vi "Begin.vi"(8 "error in":errorcluster) -> (0 "error out":errorcluster)   [LabVIEW 2018]
doc: "Called before other user functions, this VI is expected to open initial I/O refnums, load in file data, and do all program initialization. Notice that the <B>error out</B> terminal is simply used for data flow. Wiring it to other structures or subVIs ensures that this VI runs first."
uses:
  <vilib>/Rock Robotics/WPI/ThirdParty/Phoenix-LabVIEW/Motor Controller/Controls/CTRE_Phoenix_MotorControl_EnhancedMotorControllerConfigurables.ctl
  <vilib>/Rock Robotics/WPI/ThirdParty/Phoenix-LabVIEW/Motor Controller/Controls/CTRE_Phoenix_MotorControl_BaseConfigurables.ctl
  <vilib>/Rock Robotics/WPI/ThirdParty/Phoenix-LabVIEW/Motor Controller/Controls/CTRE_Phoenix_MotorControl_VelocityMeasurementPeriod.ctl
  <vilib>/Rock Robotics/WPI/ThirdParty/Phoenix-LabVIEW/Motor Controller/Controls/CTRE_Phoenix_MotorControl_SlotStructure.ctl
  <vilib>/Rock Robotics/WPI/ThirdParty/Phoenix-LabVIEW/Motor Controller/Controls/CTRE_Phoenix_MotorControl_FilterStruct.ctl
  <vilib>/Rock Robotics/WPI/ThirdParty/Phoenix-LabVIEW/Motor Controller/Controls/CTRE_Phoenix_MotorControl_RemoteSourceType.ctl
  <vilib>/Rock Robotics/WPI/ThirdParty/Phoenix-LabVIEW/Controls/CTRE_Phoenix_CustomParamConfiguration.ctl
  <vilib>/Rock Robotics/WPI/ThirdParty/Phoenix-LabVIEW/Motor Controller/Controls/CTRE_Phoenix_MotorControl_FeedbackDevice.ctl
  <vilib>/Rock Robotics/WPI/ThirdParty/Phoenix-LabVIEW/Motor Controller/Controls/CTRE_Phoenix_MotorControl_SensorTermFeedbackDevice_Enhanced.ctl
  <vilib>/Rock Robotics/WPI/ThirdParty/Phoenix-LabVIEW/Motor Controller/Controls/CTRE_Phoenix_MotorControl_LimitSwitchNormal.ctl
  <vilib>/Rock Robotics/WPI/ThirdParty/Phoenix-LabVIEW/Motor Controller/Controls/CTRE_Phoenix_MotorControl_LimitSwitchSource_Local.ctl
  <vilib>/Rock Robotics/WPI/ThirdParty/Phoenix-LabVIEW/Motor Controller/Controls/CTRE_Phoenix_MotorControl_MotorControllerConfigurables.ctl
  <vilib>/Rock Robotics/WPI/ThirdParty/Phoenix-LabVIEW/Motor Controller/Controls/CTRE_Phoenix_MotorControl_RemoteFeedbackDevice.ctl
  <vilib>/Rock Robotics/WPI/ThirdParty/Phoenix-LabVIEW/Motor Controller/Controls/CTRE_Phoenix_MotorControl_SensorTermFeedbackDevice.ctl
  <vilib>/Rock Robotics/WPI/ThirdParty/Phoenix-LabVIEW/Motor Controller/Controls/CTRE_Phoenix_MotorControl_LimitSwitchSource.ctl
  <vilib>/Rock Robotics/WPI/DriverStation/WPI_DriverStationRobotMode2.ctl
  <vilib>/Rock Robotics/WPI/Joystick/WPI_JoystickDeviceEnum.ctl
  <vilib>/Rock Robotics/WPI/Solenoid/WPI_SolenoidChannel.ctl
  <vilib>/Rock Robotics/SystemInterfaces/AI/FPGA_AIChannel.ctl
  <vilib>/Rock Robotics/WPI/ThirdParty/Phoenix-LabVIEW/Motor Controller/Controls/CTRE_Phoenix_MotorControl_NeutralMode.ctl
  <vilib>/Rock Robotics/WPI/SafetyOutput/WPI_SafetyOutputConfigMenu.ctl
  <vilib>/Rock Robotics/WPI/Accelerometer/WPI_AccelerometerRange.ctl
  <vilib>/Rock Robotics/WPI/ThirdParty/REV Robotics/SPARK MAX/Typedef/Spark MAX Idle Mode.ctl
  <vilib>/Rock Robotics/SystemInterfaces/DIO/FPGA_DIOPWMChannel.ctl
  Robot Global Data.vi
  RefNums_DriverStation.vi
  <vilib>/Rock Robotics/Network Tables/NT Write String Array.vi
  <vilib>/Rock Robotics/WPI/Solenoid/WPI_SolenoidOpenDouble.vi
  RefNums_Actuators.vi
  <vilib>/Rock Robotics/WPI/Utilities/WPI_GetSetVariantRefNum.vi
  RefNums_Sensors.vi
  <vilib>/Rock Robotics/WPI/Accelerometer/InternalAccelerometer/WPI_AccelerometerInternalOpen.vi
  <vilib>/Rock Robotics/WPI/Solenoid/WPI_SolenoidOpenSingle.vi
  <vilib>/Rock Robotics/WPI/RobotDrive/WPI_RobotDriveOpen4MotorWithExistingMotors.vi
panel:
  in  "Victor Enhanced Control":T1={"Base Configurables"={"openLoopRamp"=0.0, "closedLoopRamp"=0.0, "peakOutputForward"=1.0, "peakOutputReverse"=-1.0, "nominalOutputForward"=0.0, "nominalOutputReverse"=0.0, "neutralDeadband"=0.04, "voltageCompSaturation"=0.0, "voltageMeasurementFilter"=32, "velocityMeasurementPeriod"=100, "velocityMeasurementWindow"=64, "forwardSoftLimitThreshold"=0, "reverseSoftLimitThreshold"=0, "forwardSoftLimitEnable"=FALSE, "reverseSoftLimitEnable"=FALSE, "slot0"={"P"=0.0, "I"=0.0, "D"=0.0, "F"=0.0, "integralZone"=0.0, "allowableClosedLoopError"=0, "maxIntegralAccumulator"=0.0, "closedLoopPeakOutput"=1.0, "closedLoopPeriod"=1}, "slot1"={"P"=0.0, "I"=0.0, "D"=0.0, "F"=0.0, "integralZone"=0.0, "allowableClosedLoopError"=0, "maxIntegralAccumulator"=0.0, "closedLoopPeakOutput"=1.0, "closedLoopPeriod"=1}, "slot2"={"P"=0.0, "I"=0.0, "D"=0.0, "F"=0.0, "integralZone"=0.0, "allowableClosedLoopError"=0, "maxIntegralAccumulator"=0.0, "closedLoopPeakOutput"=1.0, "closedLoopPeriod"=1}, "slot3"={"P"=0.0, "I"=0.0, "D"=0.0, "F"=0.0, "integralZone"=0.0, "allowableClosedLoopError"=0, "maxIntegralAccumulator"=0.0, "closedLoopPeakOutput"=1.0, "closedLoopPeriod"=1}, "auxPIDPolarity"=FALSE, "remoteFilter0"={"remoteSensorDeviceID"=0, "remoteSensorSource"=enum."Off"}, "remoteFilter1"={"remoteSensorDeviceID"=0, "remoteSensorSource"=enum."Off"}, "motionCruiseVelocity"=0, "motionAcceleration"=0, "motionProfileTrajectoryPeriod"=0, "feedbackNotContinuous"=FALSE, "remoteSensorClosedLoopDisableNeutralOnLOS"=FALSE, "clearPositionOnLimitF"=FALSE, "clearPositionOnLimitR"=FALSE, "clearPositionOnQuadIdx"=FALSE, "limitSwitchDisableNeutralOnLOS"=FALSE, "softLimitDisableNeutralOnLOS"=FALSE, "pulseWidthPeriod_EdgesPerRot"=1, "pulseWidthPeriod_FilterWindowSz"=1, "customParam"={"customParam0"=0, "customParam1"=0}, "trajectoryInterpolationEnable"=TRUE}, "primaryPID"={"selectedFeedbackCoefficient"=1.0, "selectedFeedbackSensor"=11}, "auxiliaryPID"={"selectedFeedbackCoefficient"=1.0, "selectedFeedbackSensor"=11}, "sum 0 term"=11, "sum 1 term"=11, "diff 0 term "=11, "diff 1 term"=11, "forwardLimitSwitchDeviceID"=0, "reverseLimitSwitchDeviceID"=0, "forwardLimitSwitchNormal"=enum."Normally Open", "reverseLimitSwitchNormal"=enum."Normally Open", "forwardLimitSwitchSource"=3, "reverseLimitSwitchSource"=3} {"diff 1 term" items=["Remote Source 0"=11, "Remote Source 1"=12, "Software Emulated"=15]; "diff 0 term" items=["Remote Source 0"=11, "Remote Source 1"=12, "Software Emulated"=15]; "sum 1 term" items=["Remote Source 0"=11, "Remote Source 1"=12, "Software Emulated"=15]; "sum 0 term" items=["Remote Source 0"=11, "Remote Source 1"=12, "Software Emulated"=15]; "reverseLimitSwitchSource" items=["Remote Talon SRX"=1, "Remote CANifier"=2, "Deactivated"=3]; "forwardLimitSwitchSource" items=["Remote Talon SRX"=1, "Remote CANifier"=2, "Deactivated"=3]; "auxiliaryPID"."selectedFeedbackSensor" items=["Sensor Sum (S0 + S1)"=9, "Sensor Difference (D0 - D1)"=10, "Remote Source 0"=11, "Remote Source 1"=12, "Software Emulated"=15]; "primaryPID"."selectedFeedbackSensor" items=["Sensor Sum (S0 + S1)"=9, "Sensor Difference (D0 - D1)"=10, "Remote Source 0"=11, "Remote Source 1"=12, "Software Emulated"=15]; "Base Configurables"."velocityMeasurementPeriod" items=["Period_1ms"=1, "Period_2ms"=2, "Period_5ms"=5, "Period_10ms"=10, "Period_20ms"=20, "Period_25ms"=25, "Period_50ms"=50, "Period_100ms"=100]}
  in  "Talon Enhanced Config":T12={"Base Configurables"={"openLoopRamp"=0.0, "closedLoopRamp"=0.0, "peakOutputForward"=1.0, "peakOutputReverse"=-1.0, "nominalOutputForward"=0.0, "nominalOutputReverse"=0.0, "neutralDeadband"=0.04, "voltageCompSaturation"=0.0, "voltageMeasurementFilter"=32, "velocityMeasurementPeriod"=100, "velocityMeasurementWindow"=64, "forwardSoftLimitThreshold"=0, "reverseSoftLimitThreshold"=0, "forwardSoftLimitEnable"=FALSE, "reverseSoftLimitEnable"=FALSE, "slot0"={"P"=0.0, "I"=0.0, "D"=0.0, "F"=0.0, "integralZone"=0.0, "allowableClosedLoopError"=0, "maxIntegralAccumulator"=0.0, "closedLoopPeakOutput"=1.0, "closedLoopPeriod"=1}, "slot1"={"P"=0.0, "I"=0.0, "D"=0.0, "F"=0.0, "integralZone"=0.0, "allowableClosedLoopError"=0, "maxIntegralAccumulator"=0.0, "closedLoopPeakOutput"=1.0, "closedLoopPeriod"=1}, "slot2"={"P"=0.0, "I"=0.0, "D"=0.0, "F"=0.0, "integralZone"=0.0, "allowableClosedLoopError"=0, "maxIntegralAccumulator"=0.0, "closedLoopPeakOutput"=1.0, "closedLoopPeriod"=1}, "slot3"={"P"=0.0, "I"=0.0, "D"=0.0, "F"=0.0, "integralZone"=0.0, "allowableClosedLoopError"=0, "maxIntegralAccumulator"=0.0, "closedLoopPeakOutput"=1.0, "closedLoopPeriod"=1}, "auxPIDPolarity"=FALSE, "remoteFilter0"={"remoteSensorDeviceID"=0, "remoteSensorSource"=enum."Off"}, "remoteFilter1"={"remoteSensorDeviceID"=0, "remoteSensorSource"=enum."Off"}, "motionCruiseVelocity"=0, "motionAcceleration"=0, "motionProfileTrajectoryPeriod"=0, "feedbackNotContinuous"=FALSE, "remoteSensorClosedLoopDisableNeutralOnLOS"=FALSE, "clearPositionOnLimitF"=FALSE, "clearPositionOnLimitR"=FALSE, "clearPositionOnQuadIdx"=FALSE, "limitSwitchDisableNeutralOnLOS"=FALSE, "softLimitDisableNeutralOnLOS"=FALSE, "pulseWidthPeriod_EdgesPerRot"=1, "pulseWidthPeriod_FilterWindowSz"=1, "customParam"={"customParam0"=0, "customParam1"=0}, "trajectoryInterpolationEnable"=TRUE}, "primaryPID"={"selectedFeedbackCoefficient"=1.0, "selectedFeedbackSensor"=0}, "auxiliaryPID"={"selectedFeedbackCoefficient"=1.0, "selectedFeedbackSensor"=0}, "sum0Term"=0, "sum1Term"=0, "diff0Term"=0, "diff1Term"=0, "forwardLimitSwitchNormal"=enum."Normally Open", "reverseLimitSwitchNormal"=enum."Normally Open", "forwardLimitSwitchDeviceID"=0, "reverseLimitSwitchDeviceID"=0, "forwardLimitSwitchSource"=enum."Feedback Connector", "reverseLimitSwitchSource"=enum."Feedback Connector", "peakCurrentLimit"=1, "peakCurrentDuration"=1, "continuousCurrentLimit"=1} {"diff1Term" items=["QuadEncoder"=0, "Analog"=2, "Tachometer"=4, "Pulse Width Encoded Position"=8, "Remote Source 0"=11, "Remote Source 1"=12, "Software Emulated"=15]; "diff0Term" items=["QuadEncoder"=0, "Analog"=2, "Tachometer"=4, "Pulse Width Encoded Position"=8, "Remote Source 0"=11, "Remote Source 1"=12, "Software Emulated"=15]; "sum1Term" items=["QuadEncoder"=0, "Analog"=2, "Tachometer"=4, "Pulse Width Encoded Position"=8, "Remote Source 0"=11, "Remote Source 1"=12, "Software Emulated"=15]; "sum0Term" items=["QuadEncoder"=0, "Analog"=2, "Tachometer"=4, "Pulse Width Encoded Position"=8, "Remote Source 0"=11, "Remote Source 1"=12, "Software Emulated"=15]; "auxiliaryPID"."selectedFeedbackSensor" items=["QuadEncoder"=0, "Analog"=2, "Tachometer"=4, "Pulse Width Encoded Position"=8, "Sensor Sum (S0 + S1)"=9, "Sensor Difference (D0 - D1)"=10, "Remote Source 0"=11, "Remote Source 1"=12, "Software Emulated"=15]; "primaryPID"."selectedFeedbackSensor" items=["QuadEncoder"=0, "Analog"=2, "Tachometer"=4, "Pulse Width Encoded Position"=8, "Sensor Sum (S0 + S1)"=9, "Sensor Difference (D0 - D1)"=10, "Remote Source 0"=11, "Remote Source 1"=12, "Software Emulated"=15]; "Base Configurables"."velocityMeasurementPeriod" items=["Period_1ms"=1, "Period_2ms"=2, "Period_5ms"=5, "Period_10ms"=10, "Period_20ms"=20, "Period_25ms"=25, "Period_50ms"=50, "Period_100ms"=100]}
  # "Sum and Diff terms are ways to select more than one sensor as a feedback device. \n Sum 0 is the first feedback device to be used for the Sum term, \n Sum 1 is the feedback device to be added to Sum 0 for the Sum term\n Diff 0 and Diff 1 work in a similar manner"
  # "These are only applicable\nif using a remote limit switch.\n\nLocal limit switches/no limit\nswitches do not use this"
  # "False: Primary Output = PID[0] + PID[1]  ---  Auxiliary Output = PID[0] - PID[1]\nTrue:  Primary Output = PID[0] - PID[1] --- Auxiliary Output = PID[0] + PID[1]"
  # "Enable the motion profile executor to perform linear interpolation between profile points.  Defaults to True."
  # "Sum and Diff terms are ways to select more than one sensor as a feedback device. \n Sum 0 is the first feedback device to be used for the Sum term.\n Sum 1 is the feedback device to be added to Sum 0 for the Sum term.\n Diff 0 and Diff 1 work in a similar manner."
  # "These are only applicable\nif using a remote limit switch.\n\nLocal limit switches/no limit\nswitches do not use this."
  # "Current is below Continuous threshold AND\n\n(Requested output is weaker** than applied motor\noutput OR is in the opposite direction).\n/\nMotor output is set to requested output."
  # "Current is above Peak* Threshold for Peak Duration.\n/\nReduce motor output (towards neutral)."
  # "Current is below Continuous threshold.\n/\nRamp motor output towards requested output."
  # "Current is above Continuous threshold.\n/\nReduce motor output (towards neutral)."
  # "Current Limiting is NOT enabled\nby default.\nCall this VI to enable."
  # "*If the configured Peak Threshold is less than the Continuous Threshold, the applied Peak Threshold is set equal to the Configured Continuous Threshold in firmware.\n** Both requested output and applied motor output are in the same direction, and requested output is closer to neutral."
  # "False: Primary Output = PID[0] + PID[1]  ---  Auxiliary Output = PID[0] - PID[1]\nTrue:  Primary Output = PID[0] - PID[1] --- Auxiliary Output = PID[0] + PID[1]"
  # "Enable the motion profile executor to perform linear interpolation between profile points.  Defaults to True."
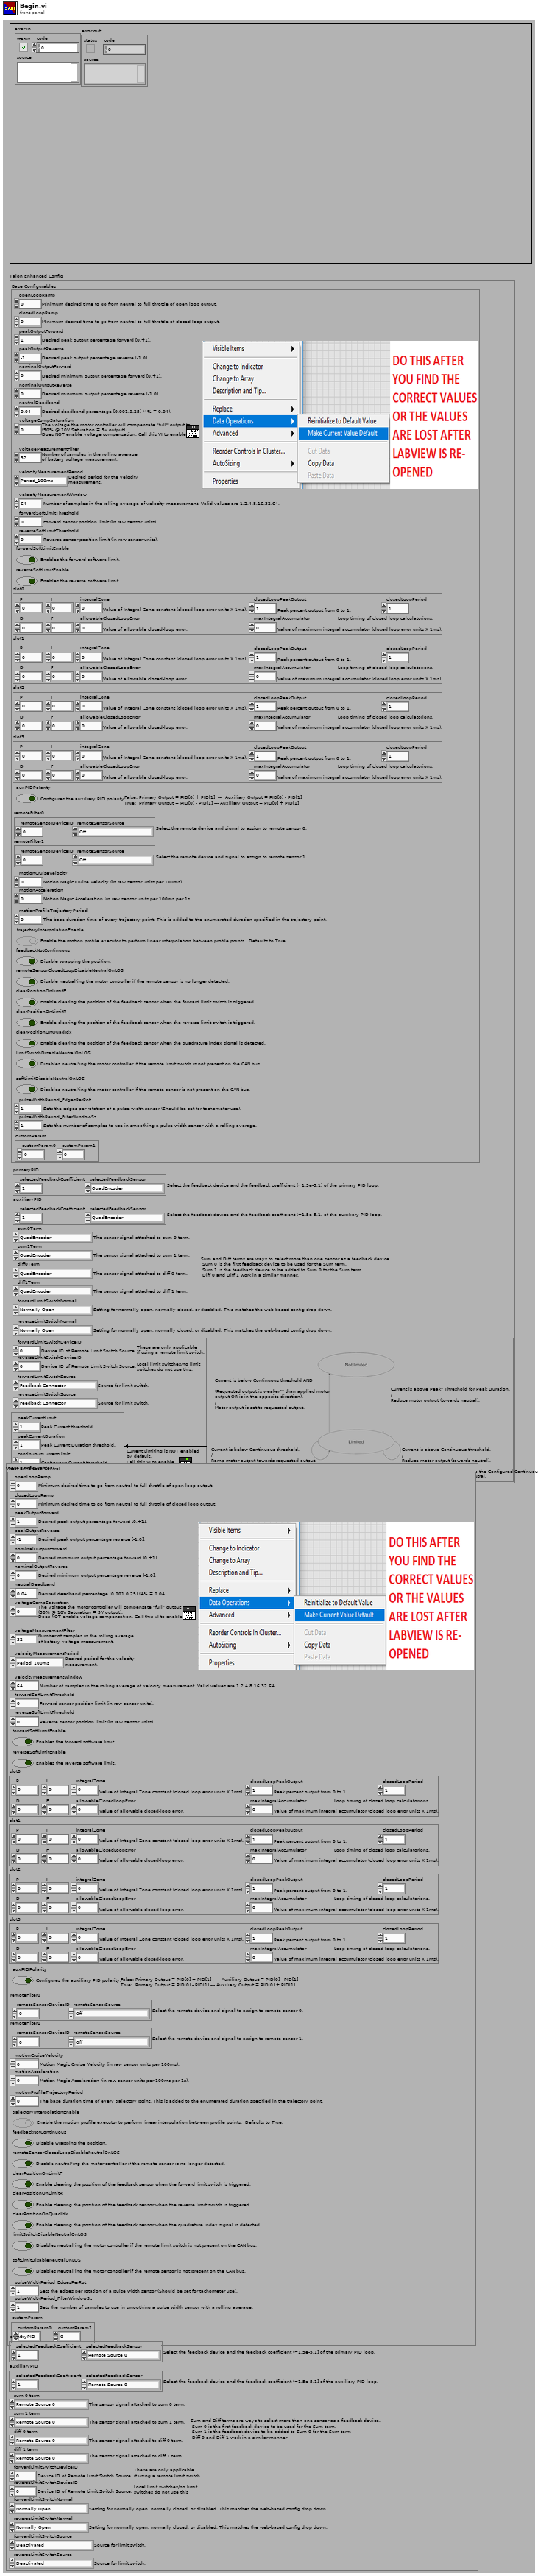
[diagram p1: front panel]
types:
  T1 = typedef "CTRE_Phoenix_MotorControl_MotorControllerConfigurables.ctl" = cluster{"Base Configurables":T2, "primaryPID":cluster{"selectedFeedbackCoefficient":dbl, "selectedFeedbackSensor":T8}, "auxiliaryPID":cluster{"selectedFeedbackCoefficient":dbl, "selectedFeedbackSensor":T8}, "sum 0 term":T9, "sum 1 term":T9, "diff 0 term ":T9, "diff 1 term":T9, "forwardLimitSwitchDeviceID":i32, "reverseLimitSwitchDeviceID":i32, "forwardLimitSwitchNormal":T10, "reverseLimitSwitchNormal":T10, "forwardLimitSwitchSource":T11, "reverseLimitSwitchSource":T11}
  T2 = typedef "CTRE_Phoenix_MotorControl_BaseConfigurables.ctl" = cluster{"openLoopRamp":dbl, "closedLoopRamp":dbl, "peakOutputForward":dbl, "peakOutputReverse":dbl, "nominalOutputForward":dbl, "nominalOutputReverse":dbl, "neutralDeadband":dbl, "voltageCompSaturation":dbl, "voltageMeasurementFilter":i32, "velocityMeasurementPeriod":T3, "velocityMeasurementWindow":i32, "forwardSoftLimitThreshold":i32, "reverseSoftLimitThreshold":i32, "forwardSoftLimitEnable":bool, "reverseSoftLimitEnable":bool, "slot0":T4, "slot1":T4, "slot2":T4, "slot3":T4, "auxPIDPolarity":bool, "remoteFilter0":T5, "remoteFilter1":T5, "motionCruiseVelocity":i32, "motionAcceleration":i32, "motionProfileTrajectoryPeriod":i32, "feedbackNotContinuous":bool, "remoteSensorClosedLoopDisableNeutralOnLOS":bool, "clearPositionOnLimitF":bool, "clearPositionOnLimitR":bool, "clearPositionOnQuadIdx":bool, "limitSwitchDisableNeutralOnLOS":bool, "softLimitDisableNeutralOnLOS":bool, "pulseWidthPeriod_EdgesPerRot":i32, "pulseWidthPeriod_FilterWindowSz":i32, "customParam":T7, "trajectoryInterpolationEnable":bool}
  T3 = typedef "CTRE_Phoenix_MotorControl_VelocityMeasurementPeriod.ctl" = u16
  T4 = typedef "CTRE_Phoenix_MotorControl_SlotStructure.ctl" = cluster{"P":dbl, "I":dbl, "D":dbl, "F":dbl, "integralZone":dbl, "allowableClosedLoopError":i32, "maxIntegralAccumulator":dbl, "closedLoopPeakOutput":dbl, "closedLoopPeriod":i32}
  T5 = typedef "CTRE_Phoenix_MotorControl_FilterStruct.ctl" = cluster{"remoteSensorDeviceID":u8, "remoteSensorSource":T6}
  T6 = typedef "CTRE_Phoenix_MotorControl_RemoteSourceType.ctl" = enum16{"Off", "Talon SRX Selected Sensor", "Pigeon IMU Yaw", "Pigeon IMU Pitch", "Pigeon IMU Roll", "CANifier Quadrature", "CANifier PWM Input 0", "CANifier PWM Input 1", "CANifier PWM Input 2", "CANifier PWM Input 3", "Gadgeteer Pigeon Yaw", "Gadgeteer Pigeon Pitch", "Gadgeteer Pigeon Roll"}
  T7 = typedef "CTRE_Phoenix_CustomParamConfiguration.ctl" = cluster{"customParam0":i32, "customParam1":i32}
  T8 = typedef "CTRE_Phoenix_MotorControl_RemoteFeedbackDevice.ctl" = i8
  T9 = typedef "CTRE_Phoenix_MotorControl_SensorTermFeedbackDevice.ctl" = i8
  T10 = typedef "CTRE_Phoenix_MotorControl_LimitSwitchNormal.ctl" = enum16{"Normally Open", "Normally Closed", "Disabled"}
  T11 = typedef "CTRE_Phoenix_MotorControl_LimitSwitchSource.ctl" = u16
  T12 = typedef "CTRE_Phoenix_MotorControl_EnhancedMotorControllerConfigurables.ctl" = cluster{"Base Configurables":T2, "primaryPID":cluster{"selectedFeedbackCoefficient":dbl, "selectedFeedbackSensor":T13}, "auxiliaryPID":cluster{"selectedFeedbackCoefficient":dbl, "selectedFeedbackSensor":T13}, "sum0Term":T14, "sum1Term":T14, "diff0Term":T14, "diff1Term":T14, "forwardLimitSwitchNormal":T10, "reverseLimitSwitchNormal":T10, "forwardLimitSwitchDeviceID":i32, "reverseLimitSwitchDeviceID":i32, "forwardLimitSwitchSource":T15, "reverseLimitSwitchSource":T15, "peakCurrentLimit":i32, "peakCurrentDuration":i32, "continuousCurrentLimit":i32}
  T13 = typedef "CTRE_Phoenix_MotorControl_FeedbackDevice.ctl" = i8
  T14 = typedef "CTRE_Phoenix_MotorControl_SensorTermFeedbackDevice_Enhanced.ctl" = i8
  T15 = typedef "CTRE_Phoenix_MotorControl_LimitSwitchSource_Local.ctl" = enum16{"Feedback Connector", "Remote Talon SRX", "Remote CANifier", "Deactivated"}
  T16 = typedef "FPGA_DIOPWMChannel.ctl" = enum8{"PWM 0", "PWM 1", "PWM 2", "PWM 3", "PWM 4", "PWM 5", "PWM 6", "PWM 7", "PWM 8", "PWM 9", "PWM MXP 0", "PWM MXP 1", "PWM MXP 2", "PWM MXP 3", "PWM MXP 4", "PWM MXP 5", "PWM MXP 6", "PWM MXP 7", "PWM MXP 8", "PWM MXP 9", "Invalid"}
  T17 = typedef "Spark MAX Idle Mode.ctl" = enum16{"Coast", "Brake"}
  T18 = typedef "WPI_SolenoidChannel.ctl" = enum8{"Solenoid 0", "Solenoid 1", "Solenoid 2", "Solenoid 3", "Solenoid 4", "Solenoid 5", "Solenoid 6", "Solenoid 7", "Invalid"}
  T19 = typedef "WPI_AccelerometerRange.ctl" = enum16{"+/- 2 g", "+/- 4 g", "+/- 8 g"}
  T20 = typedef "WPI_SafetyOutputConfigMenu.ctl" = enum16{"Enable", "Disable"}
  T21 = typedef "WPI_JoystickDeviceEnum.ctl" = enum16{"USB 0", "USB 1", "USB 2", "USB 3", "USB 4", "USB 5"}
  T22 = typedef "CTRE_Phoenix_MotorControl_NeutralMode.ctl" = enum8{"EEPROMSetting", "Override to Coast", "Override to Brake"}
  T23 = typedef "FPGA_AIChannel.ctl" = enum8{"AI 0", "AI 1", "AI 2", "AI 3", "AI MXP 0", "AI MXP 1", "AI MXP 2", "AI MXP 3", "Invalid"}
  T24 = typedef "WPI_DriverStationRobotMode2.ctl" = enum16{"Autonomous Disabled", "Autonomous Enabled", "Teleop Disabled", "Teleop Enabled", "Disconnected", "Finish", "Test Disabled", "Test Enabled", "Emergency Stopped"}
  T25 = typedef "WPI_JoystickDevRef.ctl" = cluster{"Device":T21}
  T26 = typedef "WPI_SolenoidDevRef.ctl" = cluster{"DevStatus":errorcluster, "Pneumatics Control Module":u8, "Forward Solenoid Channel":T18, "Reverse Solenoid Channel":T18}
  T27 = typedef "WPI_CompressorDevRef.ctl" = cluster{"DevStatus":errorcluster, "Pneumatics Control Module":u8}
  T28 = typedef "WPI_MotorControlDeviceRef.ctl" = cluster{"DeviceStatus":errorcluster, "Type":T29, "PWM":cluster{"PWM Channel":T16, "DeadBand":T30}, "CAN":cluster{"Device Number":u8, "SetOutput VI Ref":variant, "GetOutput VI Ref":variant, "Enable VI Ref":variant, "Disable VI Ref":variant, "Data":variant}, "Invert":bool, "DIO PWM":cluster{"PWM \"Enable\" Channel":T16, "DIOChannel":T31, "PWM Rate":dbl}}
  T29 = typedef "WPI_MotorControlType.ctl" = enum16{"PWM", "CAN", "DIO PWM"}
  T30 = typedef "WPI_PWMDeadband.ctl" = cluster{"Name":string, "maxPositivePwm":i32, "minPositivePwm":i32, "centerPwm":i32, "maxNegativePwm":i32, "minNegativePwm":i32, "angularRange":u16}
  T31 = typedef "FPGA_DIOChannel.ctl" = enum8{"DIO 0", "DIO 1", "DIO 2", "DIO 3", "DIO 4", "DIO 5", "DIO 6", "DIO 7", "DIO 8", "DIO 9", "DIO MXP 0", "DIO MXP 1", "DIO MXP 2", "DIO MXP 3", "DIO MXP 4", "DIO MXP 5", "DIO MXP 6", "DIO MXP 7", "DIO MXP 8", "DIO MXP 9", "DIO MXP 10", "DIO MXP 11", "DIO MXP 12", "DIO MXP 13", "DIO MXP 14", "DIO MXP 15", "SPI Port CS1", "SPI Port CS2", "SPI Port CS3", "SPI Port MISO", "SPI Port MOSI", "Invalid"}
  T32 = typedef "WPI_RobotDriveDevRef.ctl" = cluster{"DevStatus":errorcluster, "Motors[]":T28[], "Square Inputs":bool, "Max Output":dbl}
  T33 = typedef "WPI_ServoDeviceRef.ctl" = cluster{"DeviceStatus":errorcluster, "PWM Channel":T16, "DeadBand":T30}
  T34 = typedef "WPI_AnalogChannelDevRef.ctl" = cluster{"DevStatus":errorcluster, "Analog Channel":T23}
  T35 = typedef "WPI_AccelerometerDevRef.ctl" = cluster{"DevStatus":errorcluster, "Scaling":T36, "Analog Channels":T37, "I2C Bus":T38, "SPI Bus":T39, "Accel Range":T40, "ADXL Axes":T41, "Handle":i32, "Device Address":u8, "Accel Type":enum16{"Analog", "ADXL345 I2C", "ADXL345 SPI", "Internal", "ADXL362 SPI"}}
  T36 = typedef "WPI_AccelerometerScaling.ctl" = cluster{"Gain (VoltsPerG)":dbl, "Center Voltage":dbl}
  T37 = typedef "WPI_AccelerometerAnalogChannels.ctl" = cluster{"X-Axis":T23, "Y-Axis":T23, "Z-Axis":T23}
  T38 = typedef "i2c_bus.ctl" = enum16{"I2C On-Board", "I2C MXP", "Invalid"}
  T39 = typedef "spi_bus.ctl" = enum16{"SPI On-Board, CS0", "SPI On-Board, CS1", "SPI On-Board, CS2", "SPI On-Board, CS3", "SPI MXP", "Invalid"}
  T40 = typedef "ADXL345 Range.ctl" = u8
  T41 = typedef "WPI_AccelerometerADXL345 Axes.ctl" = cluster{"X-Axis":bool, "Y-Axis":bool, "Z-Axis":bool}
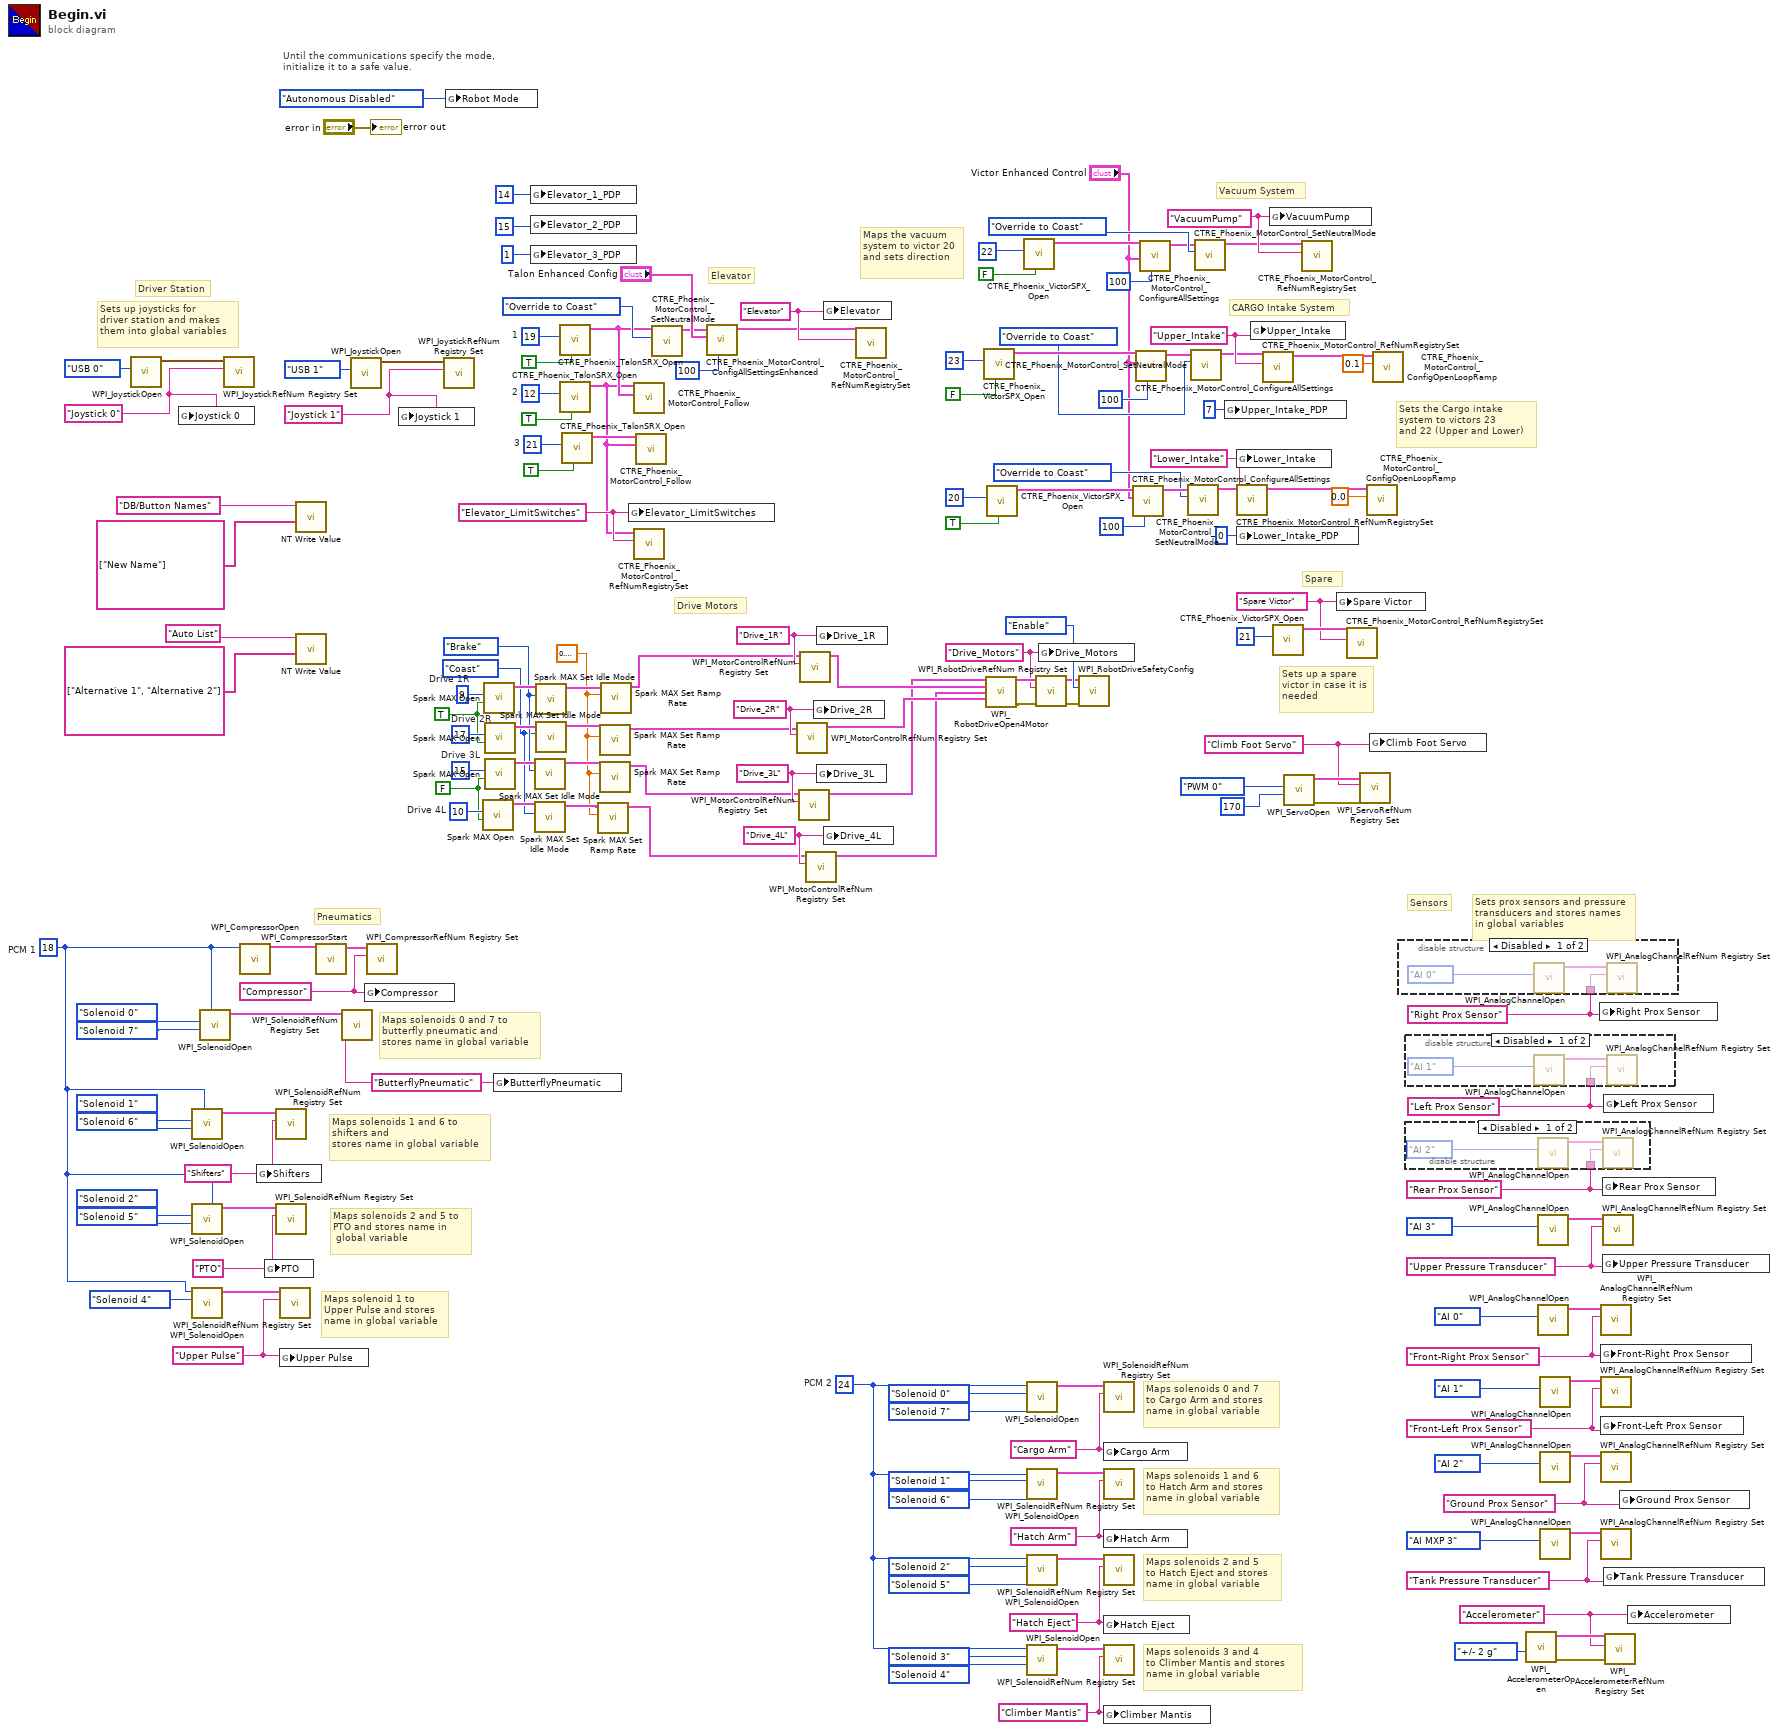
[diagram p0: block diagram]
diagram:
  w1 = "Climb Foot Servo" ("refnum name")
  w12 = sgl 0.1 ("Seconds from neutral to full (0)")
  w25 = Spark_MAX_Idle_Mode."Coast" ("Idle Mode")
  w32 = u8 21  # 3
  w35 = "Upper Pulse" ("ButterflyPneumatic")
  w26 = Spark_MAX_Idle_Mode."Brake" ("Idle Mode")
  w40 = "Accelerometer" ("refnum name")
  w44 = "Drive_4L" ("refnum name")
  w45 = "Drive_3L" ("refnum name")
  w46 = "Drive_2R" ("refnum name")
  w47 = "Drive_1R" ("refnum name")
  w48 = "Elevator_LimitSwitches" ("refnum name")
  w49 = "Drive_Motors" ("refnum name")
  w10 = FALSE ("Invert")
  w55 = u8 10  # Drive 4L
  w56 = u8 15  # Drive 3L
  w57 = u8 17  # Drive 2R
  w11 = TRUE ("Invert")
  w58 = u8 9  # Drive 1R
  w60 = "Joystick 1" ("refnum name")
  w79 = u8 12  # 2
  w84 = "Tank Pressure Transducer" ("refnum name")
  w87 = "Ground Prox Sensor" ("refnum name")
  w90 = "Front-Left Prox Sensor" ("refnum name")
  w93 = "Front-Right Prox Sensor" ("refnum name")
  w97 = "Climber Mantis" ("ButterflyPneumatic")
  w101 = "Hatch Eject" ("ButterflyPneumatic")
  w105 = "Hatch Arm" ("ButterflyPneumatic")
  w96 = u8 24  # PCM 2
  w109 = "PTO" ("ButterflyPneumatic")
  w113 = "Spare Victor" ("refnum name")
  w116 = "Upper Pressure Transducer" ("refnum name")
  w119 = "Rear Prox Sensor" ("refnum name")
  w120 = "Left Prox Sensor" ("refnum name")
  w121 = "Right Prox Sensor" ("refnum name")
  w122 = "Elevator" ("refnum name")
  w124 = u8 19  # 1
  w130 = "Lower_Intake" ("refnum name")
  w131 = "Upper_Intake" ("refnum name")
  w136 = "Cargo Arm" ("ButterflyPneumatic")
  w140 = "VacuumPump" ("refnum name")
  w143 = "Shifters" ("ButterflyPneumatic")
  w147 = "Compressor" ("Compressor")
  w148 = "ButterflyPneumatic" ("ButterflyPneumatic")
  w34 = u8 18  # PCM 1
  w154 = "Joystick 0" ("refnum name")
  # "Maps solenoid 1 to\nUpper Pulse and stores \nname in global variable"
  # "Drive Motors"
  # "Sets the Cargo intake \nsystem to victors 23 \nand 22 (Upper and Lower)"
  # "Maps the vacuum\nsystem to victor 20\nand sets direction"
  # "Sets up a spare\nvictor in case it is\nneeded"
  # "Sets up joysticks for\ndriver station and makes\nthem into global variables"
  # "Maps solenoids 3 and 4\nto Climber Mantis and stores \nname in global variable"
  # "Maps solenoids 2 and 5\nto Hatch Eject and stores \nname in global variable"
  # "Maps solenoids 1 and 6\nto Hatch Arm and stores \nname in global variable"
  # "Maps solenoids 0 and 7\nto Cargo Arm and stores \nname in global variable"
  # "Maps solenoids 2 and 5 to\nPTO and stores name in\n global variable"
  # "Maps solenoids 1 and 6 to\nshifters and \nstores name in global variable"
  # "Maps solenoids 0 and 7 to\nbutterfly pneumatic and \nstores name in global variable"
  # "Sets prox sensors and pressure\ntransducers and stores names \nin global variables"
  # "Spare"
  # "CARGO Intake System"
  # "Vacuum System"
  # "Elevator"
  # "Sensors"
  # "Pneumatics"
  # "Driver Station"
  # "Until the communications specify the mode,\ninitialize it to a safe value."
  n1 = call <vilib>:"WPI_JoystickOpen.vi"("JoystickDevice"=WPI_JoystickDeviceEnum."USB 0") -> ("JoystickDevRef"=w161:T25)  [unwired: 10 in]
  n2 = global write "RefNums_DriverStation.vi" "Joystick 0"(w154) -> ()
  n3 = call-poly <vilib>:"WPI_SolenoidOpen.vi"("Reverse Solenoid Channel"=WPI_SolenoidChannel."Solenoid 6", "Forward Solenoid Channel"=WPI_SolenoidChannel."Solenoid 1", "Pneumatics Control Module (0)"=w34) -> ("SolenoidDevRef"=w144:T26)  [unwired: 7 in, 1 out]
  n4 = call-poly <vilib>:"WPI_SolenoidOpen.vi"("Reverse Solenoid Channel"=WPI_SolenoidChannel."Solenoid 5", "Forward Solenoid Channel"=WPI_SolenoidChannel."Solenoid 2", "Pneumatics Control Module (0)"=w34) -> ("SolenoidDevRef"=w110:T26)  [unwired: 7 in, 1 out]
  n5 = call-poly <vilib>:"WPI_SolenoidOpen.vi"("Solenoid Channel"=WPI_SolenoidChannel."Solenoid 4" ("Forward Solenoid Channel"), "Pneumatics Control Module (0)"=w34) -> ("SolenoidDevRef"=w36:T26)  [unwired: 8 in, 1 out]
  n6 = call-poly <vilib>:"WPI_SolenoidOpen.vi"("Reverse Solenoid Channel"=WPI_SolenoidChannel."Solenoid 7", "Forward Solenoid Channel"=WPI_SolenoidChannel."Solenoid 0", "Pneumatics Control Module (0)"=w34) -> ("SolenoidDevRef"=w150:T26)  [unwired: 7 in, 1 out]
  n7 = call <vilib>:"WPI_JoystickRefNum Registry Set.vi"("refnum name"=w154, "JoystickDevRef"=w161) -> ()  [unwired: 8 in, 2 out]
  n8 = call <vilib>:"WPI_CompressorOpen.vi"("Pneumatics Control Module (0)"=w34) -> ("CompressorDevRef"=w153:T27)  [unwired: 13 in, 1 out]
  n9 = global write "RefNums_Actuators.vi" "Shifters"(w143) -> ()
  n10 = global write "RefNums_Actuators.vi" "PTO"(w109) -> ()
  n11 = call <vilib>:"WPI_SolenoidRefNum Registry Set.vi"("refnum name"=w143, "SolenoidDevRef"=w144) -> ()  [unwired: 8 in, 2 out]
  n12 = call <vilib>:"WPI_SolenoidRefNum Registry Set.vi"("refnum name"=w109, "SolenoidDevRef"=w110) -> ()  [unwired: 8 in, 2 out]
  n13 = call <vilib>:"WPI_SolenoidRefNum Registry Set.vi"("refnum name"=w35, "SolenoidDevRef"=w36) -> ()  [unwired: 8 in, 2 out]
  n14 = global write "RefNums_Actuators.vi" "Upper Pulse"(w35) -> ()
  n15 = call-poly <vilib>:"NT Write Value.vi"("String Array"=string[] ["New Name"], "Name"="DB/Button Names") -> ()  [unwired: 9 in, 1 out]
  n16 = call-poly <vilib>:"NT Write Value.vi"("String Array"=string[] ["Alternative 1", "Alternative 2"], "Name"="Auto List") -> ()  [unwired: 9 in, 1 out]
  n17 = call <vilib>:"WPI_CompressorStart.vi"("CompressorDevRef"=w153) -> ("CompressorDevRef"=w149:T27)  [unwired: 9 in, 1 out]
  n18 = call <vilib>:"WPI_SolenoidRefNum Registry Set.vi"("refnum name"=w148, "SolenoidDevRef"=w150) -> ()  [unwired: 8 in, 2 out]
  n19 = call <vilib>:"WPI_JoystickOpen.vi"("JoystickDevice"=WPI_JoystickDeviceEnum."USB 1") -> ("JoystickDevRef"=w59:T25)  [unwired: 10 in]
  n20 = global write "RefNums_Actuators.vi" "Compressor"(w147) -> ()
  n21 = call <vilib>:"WPI_CompressorRefNum Registry Set.vi"("refnum name"=w147, "CompressorDevRef"=w149) -> ()  [unwired: 8 in, 2 out]
  n22 = global write "RefNums_DriverStation.vi" "Joystick 1"(w60) -> ()
  n23 = call <vilib>:"WPI_JoystickRefNum Registry Set.vi"("refnum name"=w60, "JoystickDevRef"=w59) -> ()  [unwired: 8 in, 2 out]
  n24 = global write "Robot Global Data.vi" "Robot Mode"(WPI_DriverStationRobotMode2."Autonomous Disabled" ("Robot Mode")) -> ()
  n25 = call <vilib>:"Spark MAX Open.vi"("Invert"=w10, "Device Number"=w55) -> ("MotorControlDeviceRef"=w27:T28)  [unwired: 8 in, 1 out]
  n26 = call <vilib>:"Spark MAX Open.vi"("Invert"=w11, "Device Number"=w58) -> ("MotorControlDeviceRef"=w39:T28)  [unwired: 8 in, 1 out]
  n27 = call <vilib>:"Spark MAX Open.vi"("Invert"=w11, "Device Number"=w57) -> ("MotorControlDeviceRef"=w28:T28)  [unwired: 8 in, 1 out]
  n28 = call <vilib>:"Spark MAX Open.vi"("Invert"=w10, "Device Number"=w56) -> ("MotorControlDeviceRef"=w38:T28)  [unwired: 8 in, 1 out]
  n29 = global write "RefNums_Actuators.vi" "ButterflyPneumatic"(w148) -> ()
  n30 = global write "RefNums_Actuators.vi" "Elevator_1_PDP"(14 ("Lower_Intake_PDP")) -> ()
  n31 = global write "RefNums_Actuators.vi" "Elevator_2_PDP"(15 ("Lower_Intake_PDP")) -> ()
  n32 = global write "RefNums_Actuators.vi" "Elevator_3_PDP"(1 ("Lower_Intake_PDP")) -> ()
  n33 = call <vilib>:"Spark MAX Set Idle Mode.vi"("Idle Mode"=w26, "MotorControlDeviceRef in"=w38) -> ("MotorControlDeviceRef out"=w18:T28)  [unwired: 8 in, 1 out]
  n34 = call <vilib>:"Spark MAX Set Idle Mode.vi"("Idle Mode"=w25, "MotorControlDeviceRef in"=w27) -> ("MotorControlDeviceRef out"=w19:T28)  [unwired: 8 in, 1 out]
  n35 = call <vilib>:"Spark MAX Set Idle Mode.vi"("Idle Mode"=w26, "MotorControlDeviceRef in"=w39) -> ("MotorControlDeviceRef out"=w20:T28)  [unwired: 8 in, 1 out]
  n36 = call <vilib>:"Spark MAX Set Idle Mode.vi"("Idle Mode"=w25, "MotorControlDeviceRef in"=w28) -> ("MotorControlDeviceRef out"=w17:T28)  [unwired: 8 in, 1 out]
  n37 = call <vilib>:"CTRE_Phoenix_TalonSRX_Open.vi"("Invert"=TRUE, "Device Number"=w124) -> ("CAN Talon SRX Ref"=w33:T28)  [unwired: 8 in, 1 out]
  n38 = call <vilib>:"CTRE_Phoenix_TalonSRX_Open.vi"("Invert"=TRUE, "Device Number"=w79) -> ("CAN Talon SRX Ref"=w29:T28)  [unwired: 8 in, 1 out]
  n39 = call <vilib>:"CTRE_Phoenix_TalonSRX_Open.vi"("Invert"=TRUE, "Device Number"=w32) -> ("CAN Talon SRX Ref"=w30:T28)  [unwired: 8 in, 1 out]
  n40 = call <vilib>:"Spark MAX Set Ramp Rate.vi"("Seconds from neutral to full (0)"=w12, "MotorControlDeviceRef in"=w19) -> ("MotorControlDeviceRef"=w13:T28)  [unwired: 8 in, 1 out]
  n41 = call <vilib>:"Spark MAX Set Ramp Rate.vi"("Seconds from neutral to full (0)"=w12, "MotorControlDeviceRef in"=w17) -> ("MotorControlDeviceRef"=w15:T28)  [unwired: 8 in, 1 out]
  n42 = call <vilib>:"Spark MAX Set Ramp Rate.vi"("Seconds from neutral to full (0)"=w12, "MotorControlDeviceRef in"=w18) -> ("MotorControlDeviceRef"=w14:T28)  [unwired: 8 in, 1 out]
  n43 = call <vilib>:"Spark MAX Set Ramp Rate.vi"("Seconds from neutral to full (0)"=w12, "MotorControlDeviceRef in"=w20) -> ("MotorControlDeviceRef"=w16:T28)  [unwired: 8 in, 1 out]
  n44 = global write "RefNums_Actuators.vi" "Elevator_LimitSwitches"(w48) -> ()
  n45 = call <vilib>:"CTRE_Phoenix_MotorControl_Follow.vi"("Master Controller to Follow"=w33, "PhoenixMotorControlDevRef"=w29) -> ()  [unwired: 8 in, 2 out]
  n46 = call <vilib>:"CTRE_Phoenix_MotorControl_RefNumRegistrySet.vi"("refnum name"=w48, "PhoenixMotorControlDevRef"=w29) -> ()  [unwired: 8 in, 2 out]
  n47 = call <vilib>:"CTRE_Phoenix_MotorControl_Follow.vi"("Master Controller to Follow"=w29, "PhoenixMotorControlDevRef"=w30) -> ()  [unwired: 8 in, 2 out]
  n48 = call <vilib>:"CTRE_Phoenix_MotorControl_SetNeutralMode.vi"("Motor Control Neutral Mode"=CTRE_Phoenix_MotorControl_NeutralMode."Override to Coast", "PhoenixMotorControlDevRef"=w33) -> ("PhoenixMotorControlDevRef"=w82:T28)  [unwired: 8 in, 1 out]
  n49 = call <vilib>:"CTRE_Phoenix_MotorControl_ConfigAllSettingsEnhanced.vi"("timeoutMs"=100, "Enhanced Motor Controller Configurables"="Talon Enhanced Config", "PhoenixMotorControlDevRef"=w82) -> ("PhoenixMotorControlDevRef"=w81:T28)  [unwired: 7 in, 1 out]
  n50 = call <vilib>:"WPI_MotorControlRefNum Registry Set.vi"("refnum name"=w46, "MotorControlDevRef"=w15) -> ("MotorControlDevRef"=w23:T28)  [unwired: 8 in, 1 out]
  n51 = call <vilib>:"WPI_MotorControlRefNum Registry Set.vi"("refnum name"=w45, "MotorControlDevRef"=w14) -> ("MotorControlDevRef"=w22:T28)  [unwired: 8 in, 1 out]
  n52 = call <vilib>:"WPI_MotorControlRefNum Registry Set.vi"("refnum name"=w47, "MotorControlDevRef"=w16) -> ("MotorControlDevRef"=w24:T28)  [unwired: 8 in, 1 out]
  n53 = call <vilib>:"WPI_MotorControlRefNum Registry Set.vi"("refnum name"=w44, "MotorControlDevRef"=w13) -> ("MotorControlDevRef"=w21:T28)  [unwired: 8 in, 1 out]
  n54 = global write "RefNums_Actuators.vi" "Drive_2R"(w46) -> ()
  n55 = global write "RefNums_Actuators.vi" "Drive_1R"(w47) -> ()
  n56 = global write "RefNums_Actuators.vi" "Drive_3L"(w45) -> ()
  n57 = global write "RefNums_Actuators.vi" "Elevator"(w122) -> ()
  n58 = global write "RefNums_Actuators.vi" "Drive_4L"(w44) -> ()
  n59 = call <vilib>:"CTRE_Phoenix_MotorControl_RefNumRegistrySet.vi"("refnum name"=w122, "PhoenixMotorControlDevRef"=w81) -> ()  [unwired: 8 in, 2 out]
  n60 = call <vilib>:"CTRE_Phoenix_VictorSPX_Open.vi"("Invert"=FALSE, "Device Number"=u8 23) -> ("CAN Talon SRX Ref"=w67:T28)  [unwired: 8 in, 1 out]
  n61 = call-poly <vilib>:"WPI_RobotDriveOpen4Motor.vi"("Rear Left Motor Dev Ref"=w22, "Rear Right Motor Dev Ref"=w24, "Front Left Motor Dev Ref"=w21, "Front Right Motor Dev Ref"=w23) -> ("RobotDriveDevRef"=w51:T32, "error out"=w50:errorcluster)  [unwired: 10 in]
  n62 = call <vilib>:"CTRE_Phoenix_VictorSPX_Open.vi"("Invert"=TRUE, "Device Number"=u8 20) -> ("CAN Talon SRX Ref"=w66:T28)  [unwired: 8 in, 1 out]
  n63 = call <vilib>:"CTRE_Phoenix_VictorSPX_Open.vi"("Invert"=FALSE, "Device Number"=u8 22) -> ("CAN Talon SRX Ref"=w74:T28)  [unwired: 8 in, 1 out]
  n64 = call-poly <vilib>:"WPI_SolenoidOpen.vi"("Reverse Solenoid Channel"=WPI_SolenoidChannel."Solenoid 7", "Forward Solenoid Channel"=WPI_SolenoidChannel."Solenoid 0", "Pneumatics Control Module (0)"=w96) -> ("SolenoidDevRef"=w137:T26)  [unwired: 7 in, 1 out]
  n65 = call-poly <vilib>:"WPI_SolenoidOpen.vi"("Reverse Solenoid Channel"=WPI_SolenoidChannel."Solenoid 6", "Forward Solenoid Channel"=WPI_SolenoidChannel."Solenoid 1", "Pneumatics Control Module (0)"=w96) -> ("SolenoidDevRef"=w106:T26)  [unwired: 7 in, 1 out]
  n66 = call-poly <vilib>:"WPI_SolenoidOpen.vi"("Reverse Solenoid Channel"=WPI_SolenoidChannel."Solenoid 5", "Forward Solenoid Channel"=WPI_SolenoidChannel."Solenoid 2", "Pneumatics Control Module (0)"=w96) -> ("SolenoidDevRef"=w102:T26)  [unwired: 7 in, 1 out]
  n67 = call-poly <vilib>:"WPI_SolenoidOpen.vi"("Reverse Solenoid Channel"=WPI_SolenoidChannel."Solenoid 4", "Forward Solenoid Channel"=WPI_SolenoidChannel."Solenoid 3", "Pneumatics Control Module (0)"=w96) -> ("SolenoidDevRef"=w98:T26)  [unwired: 7 in, 1 out]
  n68 = call <vilib>:"WPI_RobotDriveRefNum Registry Set.vi"("error in (no error)"=w50, "refnum name"=w49, "RobotDriveDevRef"=w51) -> ("error out"=w52:errorcluster, "RobotDriveDevRef"=w53:T32)  [unwired: 7 in]
  n69 = global write "RefNums_Actuators.vi" "Drive_Motors"(w49) -> ()
  n70 = call <vilib>:"WPI_RobotDriveSafetyConfig.vi"("error in (no error)"=w52, "mode"=WPI_SafetyOutputConfigMenu."Enable", "RobotDriveDevRef"=w53) -> ()  [unwired: 7 in, 2 out]
  n71 = call <vilib>:"WPI_SolenoidRefNum Registry Set.vi"("refnum name"=w136, "SolenoidDevRef"=w137) -> ()  [unwired: 8 in, 2 out]
  n72 = global write "RefNums_Actuators.vi" "Cargo Arm"(w136) -> ()
  n73 = call <vilib>:"WPI_SolenoidRefNum Registry Set.vi"("refnum name"=w105, "SolenoidDevRef"=w106) -> ()  [unwired: 8 in, 2 out]
  n74 = global write "RefNums_Actuators.vi" "Hatch Arm"(w105) -> ()
  n75 = call <vilib>:"WPI_SolenoidRefNum Registry Set.vi"("refnum name"=w101, "SolenoidDevRef"=w102) -> ()  [unwired: 8 in, 2 out]
  n76 = global write "RefNums_Actuators.vi" "Hatch Eject"(w101) -> ()
  n77 = call <vilib>:"WPI_SolenoidRefNum Registry Set.vi"("refnum name"=w97, "SolenoidDevRef"=w98) -> ()  [unwired: 8 in, 2 out]
  n78 = global write "RefNums_Actuators.vi" "Climber Mantis"(w97) -> ()
  n79 = call <vilib>:"CTRE_Phoenix_MotorControl_ConfigureAllSettings.vi"("timeoutMs"=100, "Motor Controller Configurables"="Victor Enhanced Control", "PhoenixMotorControlDevRef"=w66) -> ("PhoenixMotorControlDevRef"=w69:T28)  [unwired: 7 in, 1 out]
  n80 = call <vilib>:"CTRE_Phoenix_MotorControl_ConfigureAllSettings.vi"("timeoutMs"=100, "Motor Controller Configurables"="Victor Enhanced Control", "PhoenixMotorControlDevRef"=w67) -> ("PhoenixMotorControlDevRef"=w68:T28)  [unwired: 7 in, 1 out]
  n81 = call <vilib>:"CTRE_Phoenix_MotorControl_ConfigureAllSettings.vi"("timeoutMs"=100, "Motor Controller Configurables"="Victor Enhanced Control", "PhoenixMotorControlDevRef"=w74) -> ("PhoenixMotorControlDevRef"=w75:T28)  [unwired: 7 in, 1 out]
  n82 = call <vilib>:"CTRE_Phoenix_MotorControl_SetNeutralMode.vi"("Motor Control Neutral Mode"=CTRE_Phoenix_MotorControl_NeutralMode."Override to Coast", "PhoenixMotorControlDevRef"=w69) -> ("PhoenixMotorControlDevRef"=w70:T28)  [unwired: 8 in, 1 out]
  n83 = call <vilib>:"CTRE_Phoenix_MotorControl_SetNeutralMode.vi"("Motor Control Neutral Mode"=CTRE_Phoenix_MotorControl_NeutralMode."Override to Coast", "PhoenixMotorControlDevRef"=w68) -> ("PhoenixMotorControlDevRef"=w63:T28)  [unwired: 8 in, 1 out]
  n84 = call <vilib>:"CTRE_Phoenix_MotorControl_SetNeutralMode.vi"("Motor Control Neutral Mode"=CTRE_Phoenix_MotorControl_NeutralMode."Override to Coast", "PhoenixMotorControlDevRef"=w75) -> ("PhoenixMotorControlDevRef"=w77:T28)  [unwired: 8 in, 1 out]
  n85 = global write "RefNums_Actuators.vi" "Upper_Intake_PDP"(7 ("Upper_Intake_PDP")) -> ()
  n86 = global write "RefNums_Actuators.vi" "Lower_Intake"(w130) -> ()
  n87 = call <vilib>:"CTRE_Phoenix_MotorControl_RefNumRegistrySet.vi"("refnum name"=w130, "PhoenixMotorControlDevRef"=w70) -> ("PhoenixMotorControlDevRef"=w129:T28)  [unwired: 8 in, 1 out]
  n88 = global write "RefNums_Actuators.vi" "Lower_Intake_PDP"(0 ("Lower_Intake_PDP")) -> ()
  n89 = global write "RefNums_Actuators.vi" "Upper_Intake"(w131) -> ()
  n90 = call <vilib>:"CTRE_Phoenix_MotorControl_RefNumRegistrySet.vi"("refnum name"=w131, "PhoenixMotorControlDevRef"=w63) -> ("PhoenixMotorControlDevRef"=w128:T28)  [unwired: 8 in, 1 out]
  n91 = global write "RefNums_Actuators.vi" "VacuumPump"(w140) -> ()
  n92 = call <vilib>:"CTRE_Phoenix_VictorSPX_Open.vi"("Device Number"=u8 21) -> ("CAN Talon SRX Ref"=w114:T28)  [unwired: 9 in, 1 out]
  n93 = call <vilib>:"WPI_ServoOpen.vi"("Angular Range"=u16 170, "PWM Channel"=FPGA_DIOPWMChannel."PWM 0") -> ("error out"=w5:errorcluster, "ServoDeviceRef"=w2:T33)  [unwired: 8 in]
  n94 = call <vilib>:"CTRE_Phoenix_MotorControl_RefNumRegistrySet.vi"("refnum name"=w140, "PhoenixMotorControlDevRef"=w77) -> ()  [unwired: 8 in, 2 out]
  n95 = global write "RefNums_Actuators.vi" "Spare Victor"(w113) -> ()
  n96 = call <vilib>:"CTRE_Phoenix_MotorControl_RefNumRegistrySet.vi"("refnum name"=w113, "PhoenixMotorControlDevRef"=w114) -> ()  [unwired: 8 in, 2 out]
  n97 = call <vilib>:"WPI_ServoRefNum Registry Set.vi"("error in (no error)"=w5, "refnum name"=w1, "ServoDeviceRef"=w2) -> ()  [unwired: 7 in, 2 out]
  n98 = call <vilib>:"CTRE_Phoenix_MotorControl_ConfigOpenLoopRamp.vi"("secondsFromNeutralToFull"=0.0, "PhoenixMotorControlDevRef"=w129) -> ()  [unwired: 8 in, 2 out]
  n99 = global write "RefNums_Actuators.vi" "Climb Foot Servo"(w1) -> ()
  n100 = call <vilib>:"CTRE_Phoenix_MotorControl_ConfigOpenLoopRamp.vi"("secondsFromNeutralToFull"=0.1, "PhoenixMotorControlDevRef"=w128) -> ()  [unwired: 8 in, 2 out]
  n101 = disable-structure shown="Disabled" {
    disable-tunnel: w121 -> [w164 _]
    frame Disabled {
      n102 = call <vilib>:"WPI_AnalogChannelOpen.vi"("Analog Channel"=FPGA_AIChannel."AI 0") -> ("AIDeviceRef"=w166:T34)  [unwired: 9 in, 1 out]
      n103 = call <vilib>:"WPI_AnalogChannelRefNum Registry Set.vi"("refnum name"=w164, "AIDeviceRef"=w166) -> ()  [unwired: 8 in, 2 out]
    }
    frame Enabled {
    }
  }
  n104 = disable-structure shown="Disabled" {
    disable-tunnel: w120 -> [w167 _]
    frame Disabled {
      n105 = call <vilib>:"WPI_AnalogChannelOpen.vi"("Analog Channel"=FPGA_AIChannel."AI 1") -> ("AIDeviceRef"=w169:T34)  [unwired: 9 in, 1 out]
      n106 = call <vilib>:"WPI_AnalogChannelRefNum Registry Set.vi"("refnum name"=w167, "AIDeviceRef"=w169) -> ()  [unwired: 8 in, 2 out]
    }
    frame Enabled {
    }
  }
  n107 = disable-structure shown="Disabled" {
    disable-tunnel: w119 -> [w170 _]
    frame Disabled {
      n108 = call <vilib>:"WPI_AnalogChannelOpen.vi"("Analog Channel"=FPGA_AIChannel."AI 2") -> ("AIDeviceRef"=w172:T34)  [unwired: 9 in, 1 out]
      n109 = call <vilib>:"WPI_AnalogChannelRefNum Registry Set.vi"("refnum name"=w170, "AIDeviceRef"=w172) -> ()  [unwired: 8 in, 2 out]
    }
    frame Enabled {
    }
  }
  n110 = call-poly <vilib>:"WPI_AccelerometerOpen.vi"("Accel Range"=WPI_AccelerometerRange."+/- 2 g") -> ("error out"=w42:errorcluster, "AccelerometerDevRef"=w43:T35)  [unwired: 9 in]
  n111 = call <vilib>:"WPI_AnalogChannelOpen.vi"("Analog Channel"=FPGA_AIChannel."AI 3") -> ("AIDeviceRef"=w118:T34)  [unwired: 9 in, 1 out]
  n112 = call <vilib>:"WPI_AnalogChannelOpen.vi"("Analog Channel"=FPGA_AIChannel."AI 0") -> ("AIDeviceRef"=w95:T34)  [unwired: 9 in, 1 out]
  n113 = call <vilib>:"WPI_AnalogChannelOpen.vi"("Analog Channel"=FPGA_AIChannel."AI 1") -> ("AIDeviceRef"=w92:T34)  [unwired: 9 in, 1 out]
  n114 = call <vilib>:"WPI_AnalogChannelOpen.vi"("Analog Channel"=FPGA_AIChannel."AI 2") -> ("AIDeviceRef"=w89:T34)  [unwired: 9 in, 1 out]
  n115 = call <vilib>:"WPI_AnalogChannelOpen.vi"("Analog Channel"=FPGA_AIChannel."AI MXP 3") -> ("AIDeviceRef"=w86:T34)  [unwired: 9 in, 1 out]
  n116 = global write "RefNums_Sensors.vi" "Right Prox Sensor"(w121) -> ()
  n117 = call <vilib>:"WPI_AnalogChannelRefNum Registry Set.vi"("refnum name"=w93, "AIDeviceRef"=w95) -> ()  [unwired: 8 in, 2 out]
  n118 = global write "RefNums_Sensors.vi" "Front-Right Prox Sensor"(w93) -> ()
  n119 = call <vilib>:"WPI_AnalogChannelRefNum Registry Set.vi"("refnum name"=w90, "AIDeviceRef"=w92) -> ()  [unwired: 8 in, 2 out]
  n120 = global write "RefNums_Sensors.vi" "Front-Left Prox Sensor"(w90) -> ()
  n121 = call <vilib>:"WPI_AnalogChannelRefNum Registry Set.vi"("refnum name"=w87, "AIDeviceRef"=w89) -> ()  [unwired: 8 in, 2 out]
  n122 = call <vilib>:"WPI_AnalogChannelRefNum Registry Set.vi"("refnum name"=w84, "AIDeviceRef"=w86) -> ()  [unwired: 8 in, 2 out]
  n123 = global write "RefNums_Sensors.vi" "Rear Prox Sensor"(w119) -> ()
  n124 = call <vilib>:"WPI_AnalogChannelRefNum Registry Set.vi"("refnum name"=w116, "AIDeviceRef"=w118) -> ()  [unwired: 8 in, 2 out]
  n125 = global write "RefNums_Sensors.vi" "Upper Pressure Transducer"(w116) -> ()
  n126 = global write "RefNums_Sensors.vi" "Left Prox Sensor"(w120) -> ()
  n127 = global write "RefNums_Sensors.vi" "Tank Pressure Transducer"(w84) -> ()
  n128 = call <vilib>:"WPI_AccelerometerRefNum Registry Set.vi"("error in (no error)"=w42, "refnum name"=w40, "AccelerometerDevRef"=w43) -> ()  [unwired: 7 in, 2 out]
  n129 = global write "RefNums_Sensors.vi" "Ground Prox Sensor"(w87) -> ()
  n130 = global write "RefNums_Sensors.vi" "Accelerometer"(w40) -> ()
  "error out" <- "error in"
